vi "Destroy User Events.vi"(11 "UI Template in":refnum<class "Interactor.lvclass">) -> (3 "UI Template out":refnum<class "Interactor.lvclass">)   [LabVIEW 2020, in "Interactor.lvlib" / "Interactor.lvclass"]
uses:
  Interactor.lvclass
  Interactor.lvclass/Interactor.ctl
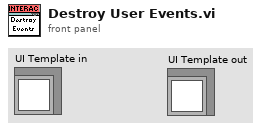
[diagram p1: front panel]
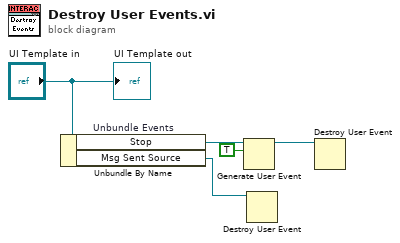
[diagram p0: block diagram]
diagram:
  n1 = Unbundle By Name "Unbundle Events"("UI Template in") -> ("Stop"=w3:refnum<user-event>, "Msg Sent Source"=w1:refnum<user-event>)
  n2 = Generate User Event(user event=w3, event data cluster=TRUE ("event data")) -> (user event out=w4:refnum<user-event>)  [unwired: 2 in, 1 out]
  n3 = Destroy User Event(user event=w1) -> ()  [unwired: 1 in, 1 out]
  n4 = Destroy User Event(user event=w4) -> ()  [unwired: 1 in, 1 out]
  "UI Template out" <- "UI Template in"
